vi "HTTP_Reply.vi"(10 "input in":string, 11 "TCP in":refnum<k5>) -> (3 "TCP out":refnum<k5>)   [LabVIEW 2020]
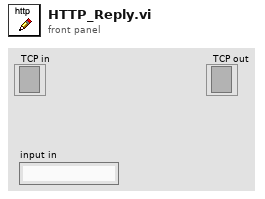
[diagram p1: front panel]
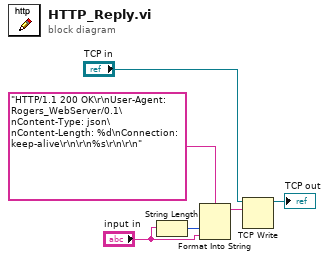
[diagram p0: block diagram]
diagram:
  n1 = String Length(string="input in") -> (length=w4:i32)
  n2 = Format Into String(format string="HTTP/1.1 200 OK\r\nUser-Agent: Rogers_WebServer/0.1\nContent-Type: json\nContent-Length: %d\nConnection: keep-alive\r\n\r\n%s\r\n\r\n" ("regular expression"), w4, "input in") -> (resulting string=w5:string)  [unwired: 2 in, 1 out]
  n3 = TCP Write(connection ID="TCP in", data in=w5) -> (connection ID out=→"TCP out":refnum<k5>)  [unwired: 2 in, 2 out]
